vi "Start Async.vi"(8 "error in (no error)":errorcluster, 11 "gRPC Server in":refnum<class "MeasurementService_Template.lvclass">) -> (0 "error out":errorcluster, 3 "gRPC Server out":refnum<class "MeasurementService_Template.lvclass">)   [LabVIEW 2020, in "MeasurementService_Template.lvlib" / "MeasurementService_Template.lvclass"]
uses:
  MeasurementService_Template.lvclass
  MeasurementService_Template.lvclass/MeasurementService_Template.ctl
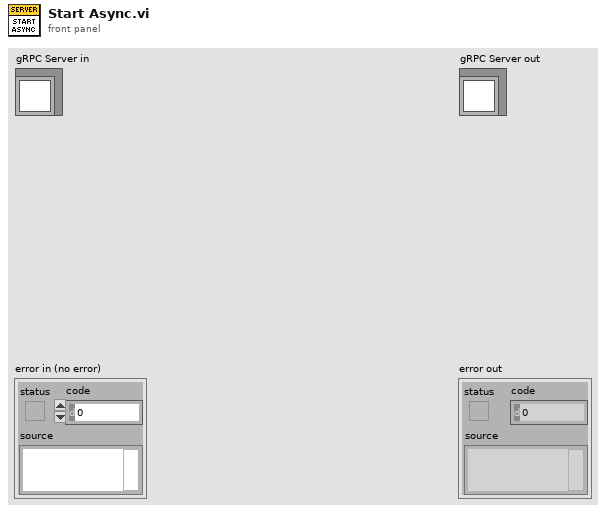
[diagram p1: front panel]
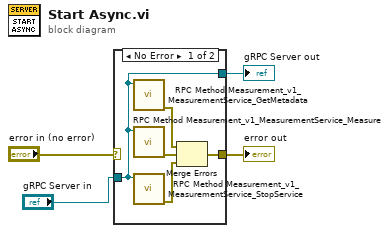
[diagram p0: block diagram]
diagram:
  n1 = case shown="No Error" "error in (no error)" {
    selector: "error in (no error)" -> [_ w11]
    tunnel: [w8 w11] -> w3
    tunnel: [w9 w10] -> w1
    tunnel: "gRPC Server in" -> [w9 w10]
    frame No Error {
      n2 = call "RPC Method Measurement_v1_MeasurementService_GetMetadata.vi"("OOP Server in"=w9) -> ("error out"=w7:errorcluster)  [unwired: 9 in, 1 out]
      n3 = call "RPC Method Measurement_v1_MeasurementService_Measure.vi"("OOP Server in"=w9) -> ("error out"=w6:errorcluster)  [unwired: 9 in, 1 out]
      n4 = call "RPC Method Measurement_v1_MeasurementService_StopService.vi"("OOP Server in"=w9) -> ("error out"=w5:errorcluster)  [unwired: 9 in, 1 out]
      n5 = Merge Errors(w7, w6, w5) -> (w8:errorcluster)
    }
    frame Error {
    }
  }
  "error out" <- w3
  "gRPC Server out" <- w1
